vi "deserialize.vi"(8 "error in":errorcluster, 10 "Flattened Waypoint":string) -> (0 "error out":errorcluster, 2 "Waypoint Out":refnum<class "Waypoint.lvclass">)   [LabVIEW 2011, in "Waypoint.lvclass"]
doc: "Deserializes a waypoint."
uses:
  Waypoint.lvclass
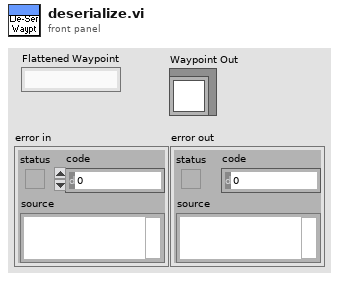
[diagram p1: front panel]
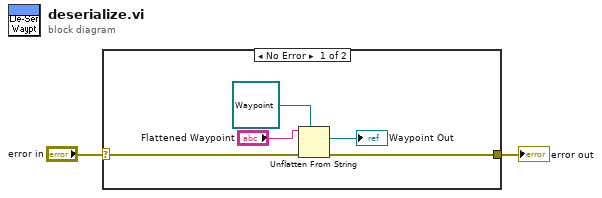
[diagram p0: block diagram]
diagram:
  n1 = case shown="No Error" "error in" {
    selector: "error in" -> [w6 w8]
    tunnel: [w7 w8] -> w2
    frame No Error {
      n2 = Unflatten From String(type=refnum<class "Waypoint.lvclass"> refnum ("Waypoint Cluster"), binary string="Flattened Waypoint", error in (no error)=w6) -> (value=→"Waypoint Out":refnum<class "Waypoint.lvclass">, error out=w7:errorcluster)  [unwired: 2 in, 1 out]
    }
    frame Error {
    }
  }
  "error out" <- w2
